vi "Generate and Broadcast Event.vi"(8 "error in (no error)":errorcluster, 10 "Event Data":refnum<class "Event.lvclass">, 11 "View in":refnum<class "View.lvclass">) -> (0 "error out":errorcluster, 3 "View out":refnum<class "View.lvclass">)   [LabVIEW 2023, in "MVC Actors.lvlib" / "View.lvclass"]
doc: "This method generates/fires the Event wired to the input. The method checks if the view is paused or \"Receive Only\" and then sends the “Generate and Broadcast Event” message to the associated controller. The controller will in turn send the Event to all the Views who registered that event but the originating View.\n\n<b>IMPORTANT</b> - Only call this method directly (i.e. without sending the corresponding message) only within the View methods. From helper loops send the corresponding message to self by calling the suitable send method. This is to make sure your View works with up-to-date settings."
uses:
  View.lvclass
  C:/Program Files/National Instruments/LabVIEW 2023/vi.lib/ActorFramework/Actor/Actor.lvclass
  Event/Event.lvclass
  View.lvclass/View.ctl
  <vilib>/ActorFramework/Actor/Actor.lvclass/Actor.ctl
  <vilib>/ActorFramework/Message Enqueuer/Message Enqueuer.lvclass/Message Enqueuer.ctl
  properties/Read Controller Actor Enqueuer.vi
  properties/Read Paused.vi
  properties/Read Receive Only.vi
  <vilib>/ActorFramework/Message Enqueuer/Init from Existing Queue.vi
  <vilib>/ActorFramework/Message Enqueuer/Message Enqueuer.lvclass
  Controller Messages/Handle and Broadcast Event Msg/Handle and Broadcast Event Msg.lvclass
  <vilib>/ActorFramework/Actor/Actor.lvclass
  C:/Projects/Shared Libraries/Event Actors/View/View.lvclass
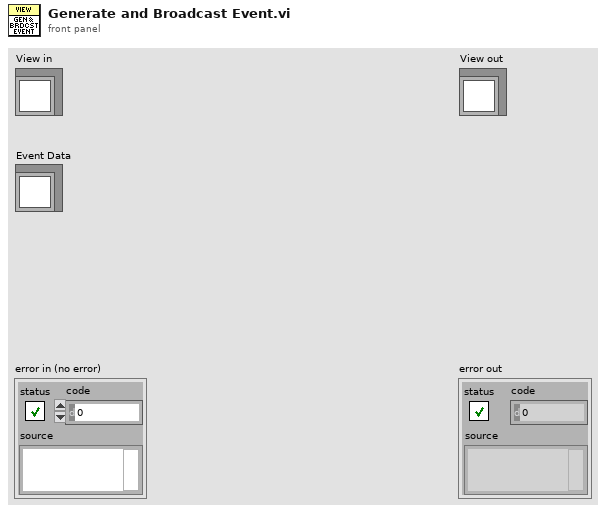
[diagram p1: front panel]
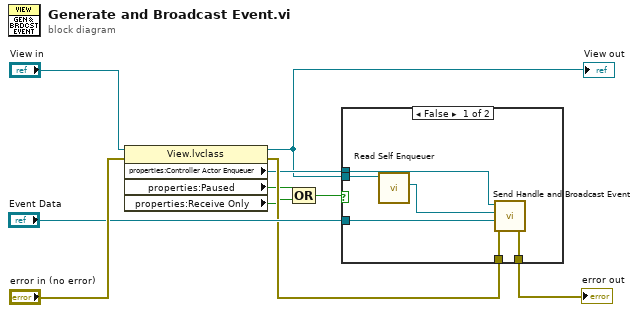
[diagram p0: block diagram]
diagram:
  n1 = property class="View.lvclass"(reference="View in", error in="error in (no error)") -> (reference out=w4:refnum<class "View.lvclass">, error out=w7:errorcluster, "properties:Controller Actor Enqueuer"=w5:refnum<class "Message Enqueuer.lvclass">, "properties:Paused"=w3:bool, "properties:Receive Only"=w2:bool)
  "View out" <- w4
  n2 = Compound Arithmetic op=OR(w3, w2) -> (w1:bool)
  n3 = case shown="False" w1 {
    tunnel: "Event Data" -> [w15 _]
    tunnel: w7 -> [w14 w17]
    tunnel: [w13 w17] -> w6
    tunnel: w5 -> [w12 _]
    tunnel: w4 -> [w11 _]
    frame False {
      n4 = call <vilib>:"Read Self Enqueuer.vi"("Actor"=w11) -> ("Self Enqueuer"=w16:refnum<class "Message Enqueuer.lvclass">)  [unwired: 10 in]
      n5 = call "Send Handle and Broadcast Event.vi"("error in (no error)"=w14, "Event Data"=w15, "View Enqueuer"=w16, "Message Enqueuer in"=w12) -> ("error out"=w13:errorcluster)  [unwired: 6 in, 1 out]
    }
    frame True {
    }
  }
  "error out" <- w6
